vi "set_addressee.vi"(8 "error in (no error)":errorcluster, 10 "addressee":string, 11 "HGF_Visitor":refnum<class "HGF_Visitor.lvclass">) -> (0 "error out":errorcluster, 3 "dup HGF_Visitor":refnum<class "HGF_Visitor.lvclass">)   [LabVIEW 2014, in "HGF_BaseClasses.lvlib" / "HGF_Visitor.lvclass"]
doc: "Set name of object that should recieve this visitor."
uses:
  HGF_Visitor.lvclass
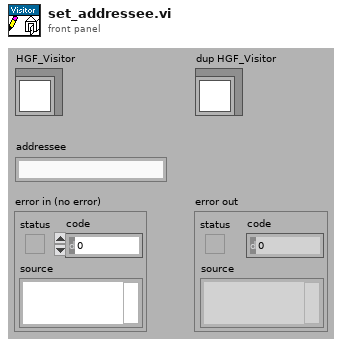
[diagram p1: front panel]
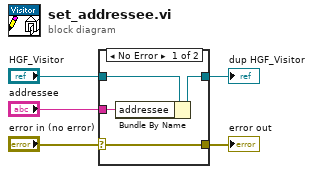
[diagram p0: block diagram]
diagram:
  n1 = case shown="No Error" "error in (no error)" {
    selector: "error in (no error)" -> [w9 w10]
    tunnel: [w9 w10] -> w4
    tunnel: [w7 w11] -> w2
    tunnel: "HGF_Visitor" -> [w8 w11]
    tunnel: "addressee" -> [w6 _]
    frame No Error {
      n2 = Bundle By Name(cluster=w8, "addressee"=w6) -> (w7:refnum<class "HGF_Visitor.lvclass">)
    }
    frame Error {
    }
  }
  "error out" <- w4
  "dup HGF_Visitor" <- w2
